vi "tcp connlimit test.vi"() -> ()   [LabVIEW 2015]
uses:
  connection/connection maintainer.lvclass
  client/connection client.lvclass/connection client.ctl
  message/communicator message.lvclass
  message/communicator message.lvclass/communicator message.ctl
  communicator/communicator.lvclass/communicator.ctl
  client/prepare client.vi
  server/prepare server.vi
  TCP/TCP server.lvclass
  TCP client/TCP client.lvclass
  communicator/communicator.lvclass
  <vilib>/ptbypt/NI_PtbyPt.lvlib
panel:
  in  "close s":bool
  in  "close c1":bool
  in  "close c2":bool
  in  "remake c 2":bool
  in  "CS 3":cluster{"ID":string, "data":string}
  in  "C to S 2":bool
  out "ClienQ 2":refnum<class "connection maintainer.lvclass">
  out "ClienT 2":timestamp
  out "data 5":variant
  out "ID 5":string
  out "data 3":variant
  out "ID 3":string
  out "data":variant
  out "ID":string
  out "Numeric":dbl
  in  "remake s":bool
  in  "remake c":bool
  in  "CS 2":cluster{"ID":string, "data":string}
  in  "CS":cluster{"ID":string, "data":string}
  in  "S to C":bool
  in  "C to S":bool
  in  "exits":bool
  out "ClienT":timestamp
  out "servT":timestamp
  out "servQ":refnum<class "connection maintainer.lvclass">
  out "ClienQ":refnum<class "connection maintainer.lvclass">
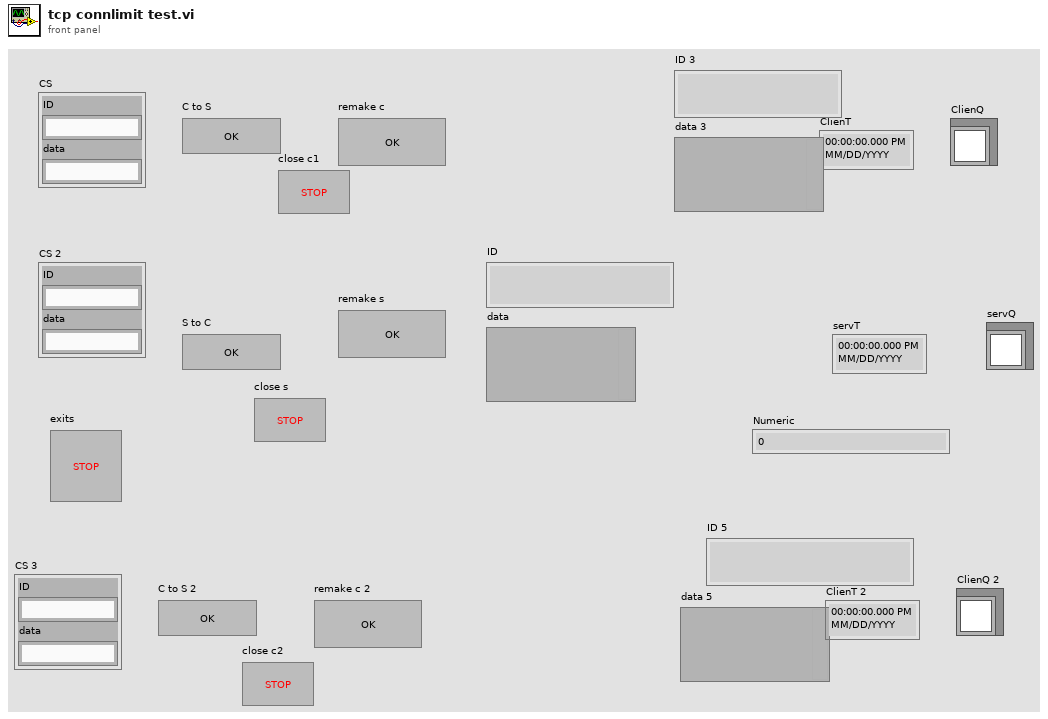
[diagram p1: front panel]
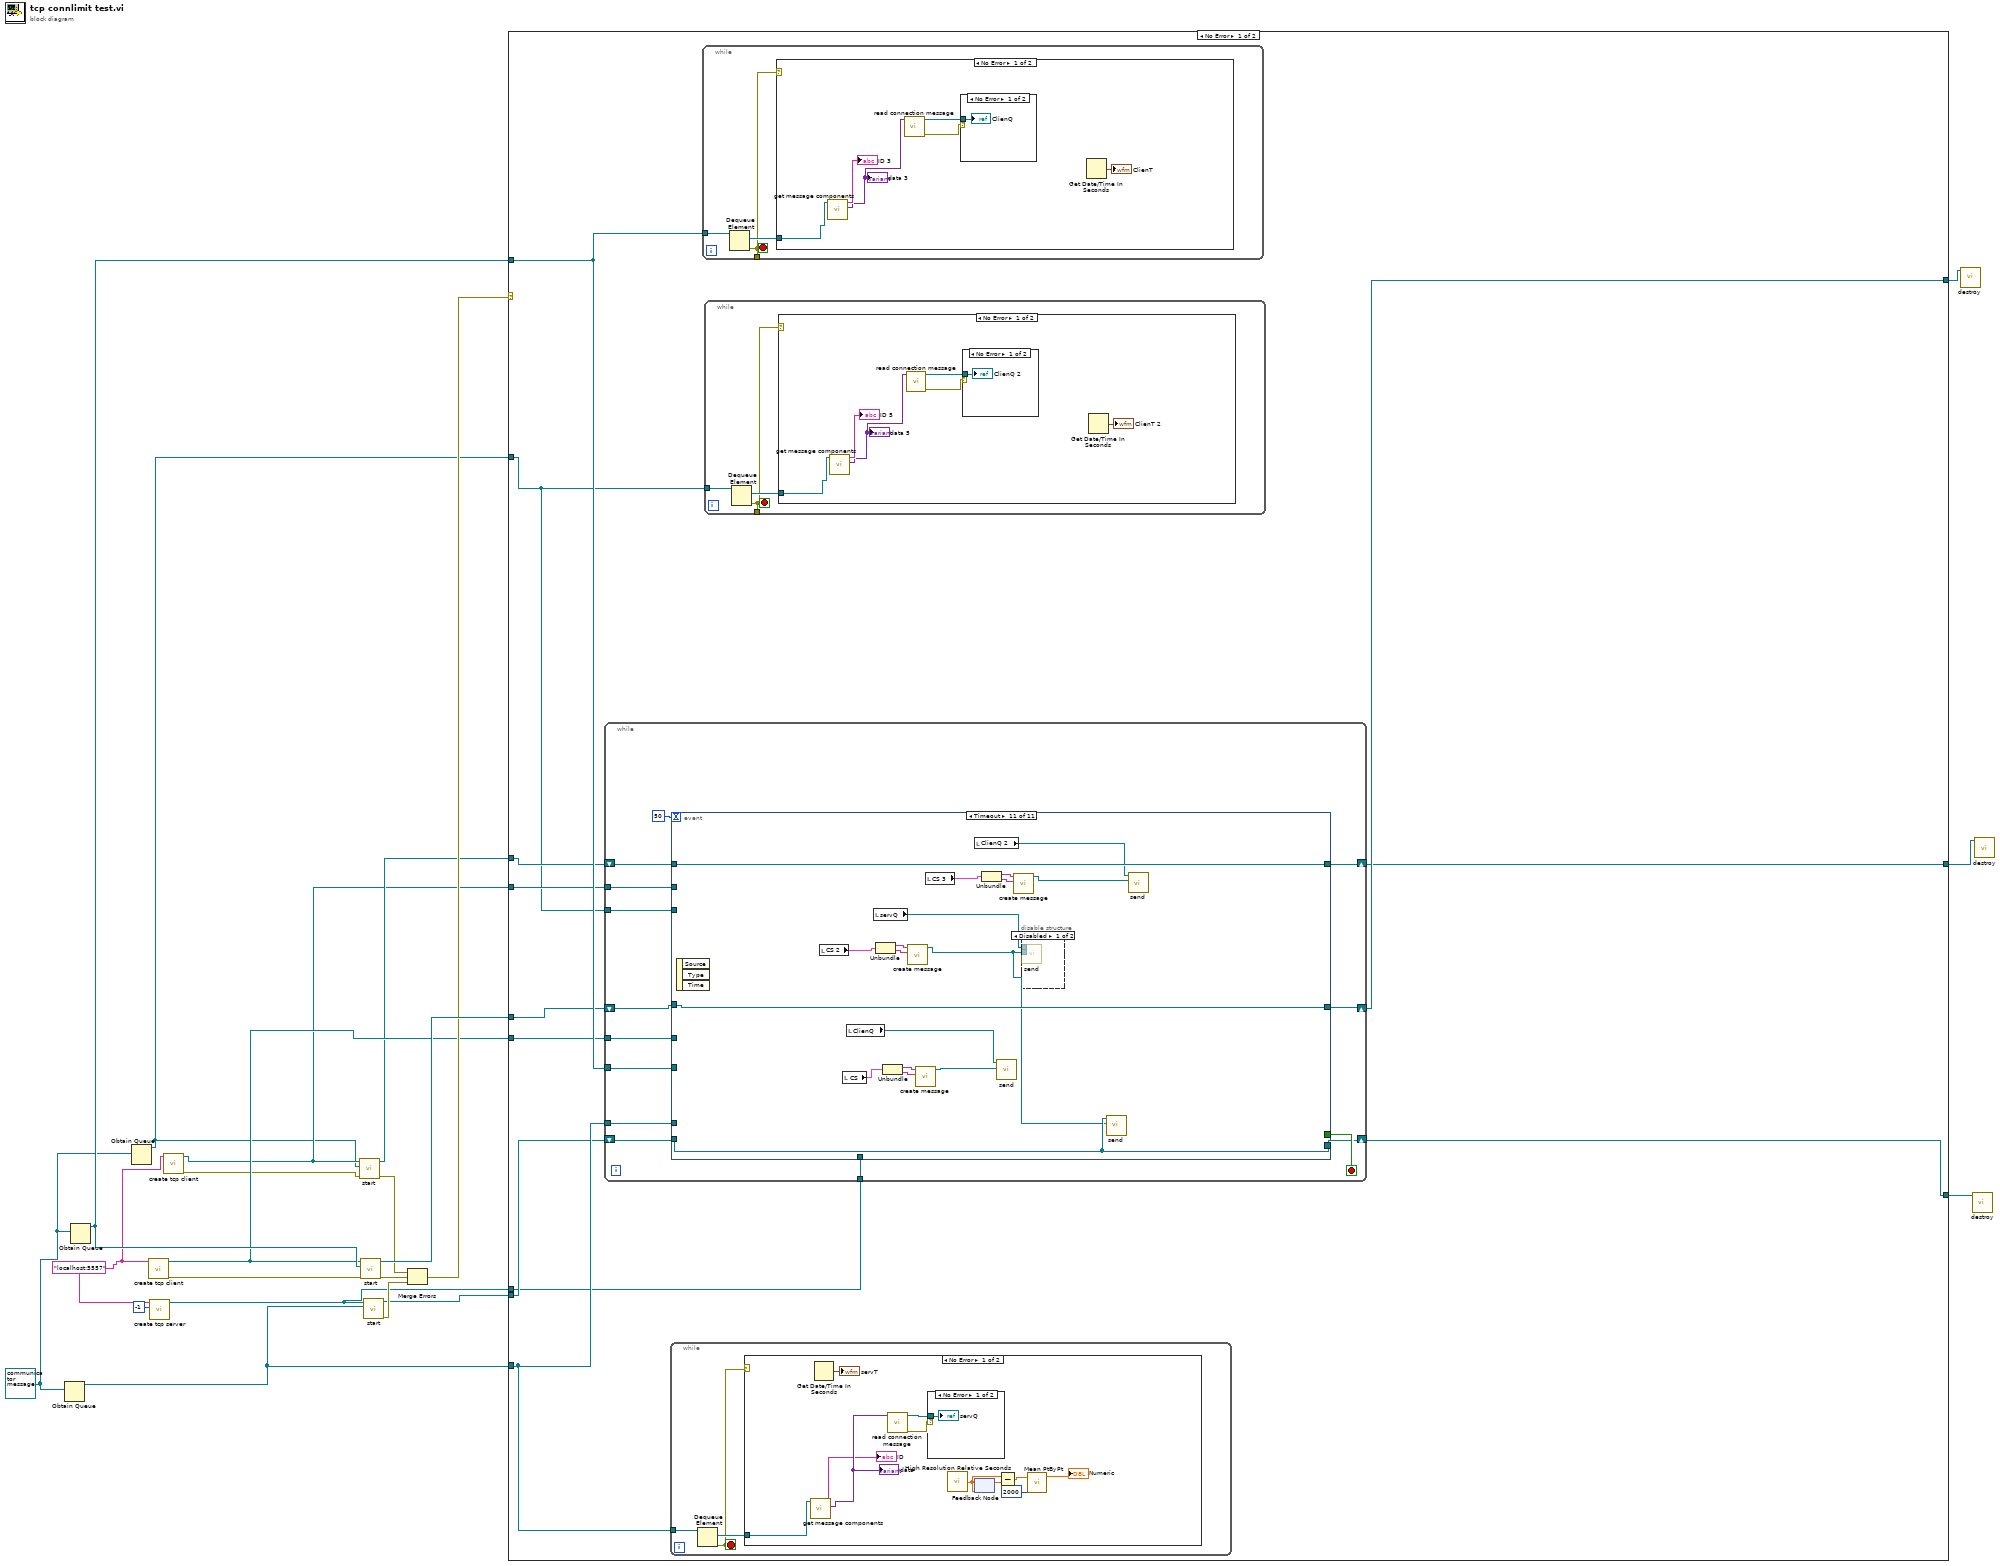
[diagram p0: block diagram]
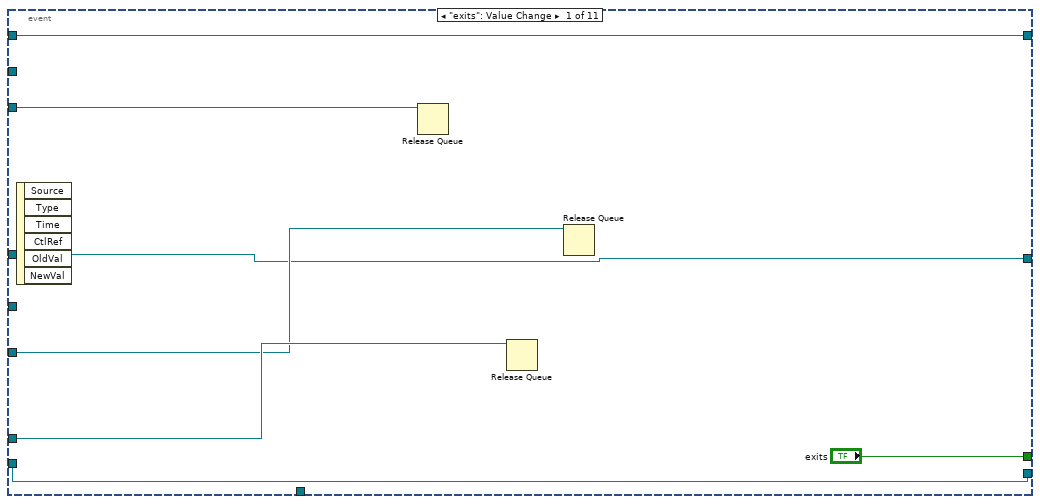
[diagram p4: hidden frame]
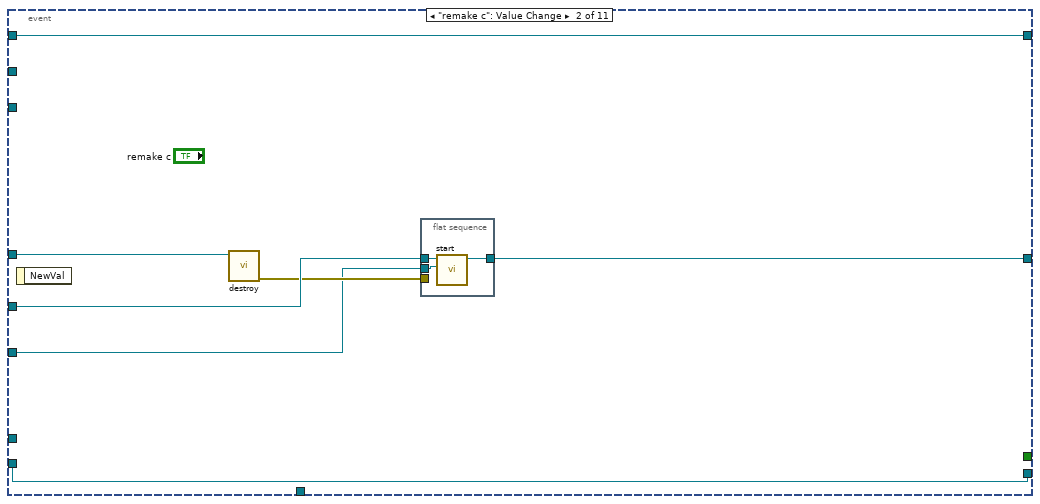
[diagram p5: hidden frame]
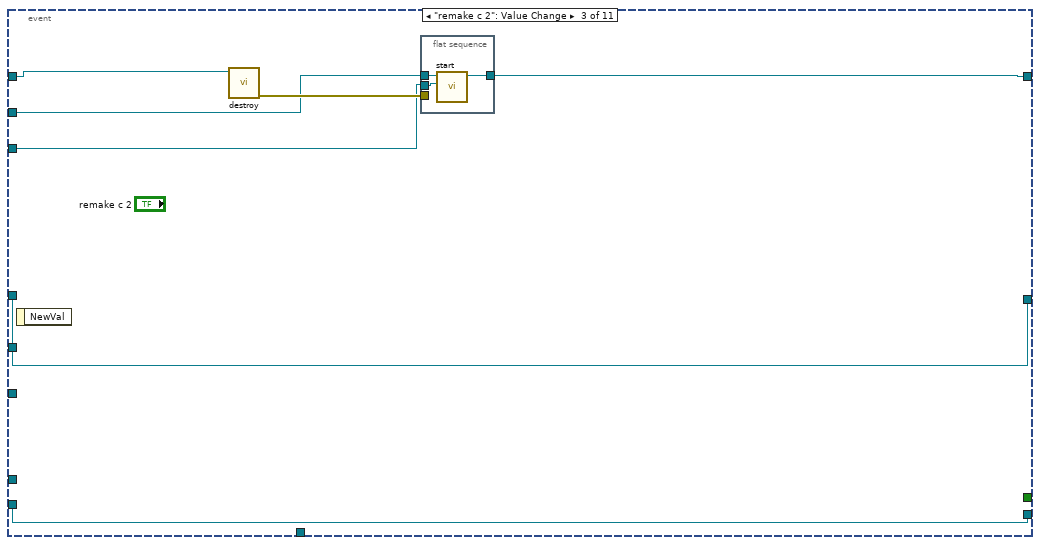
[diagram p6: hidden frame]
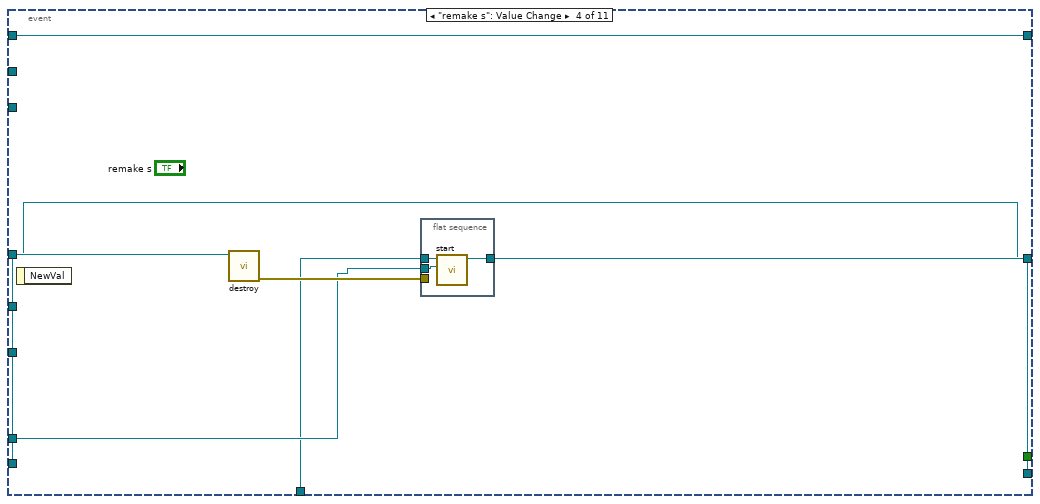
[diagram p7: hidden frame]
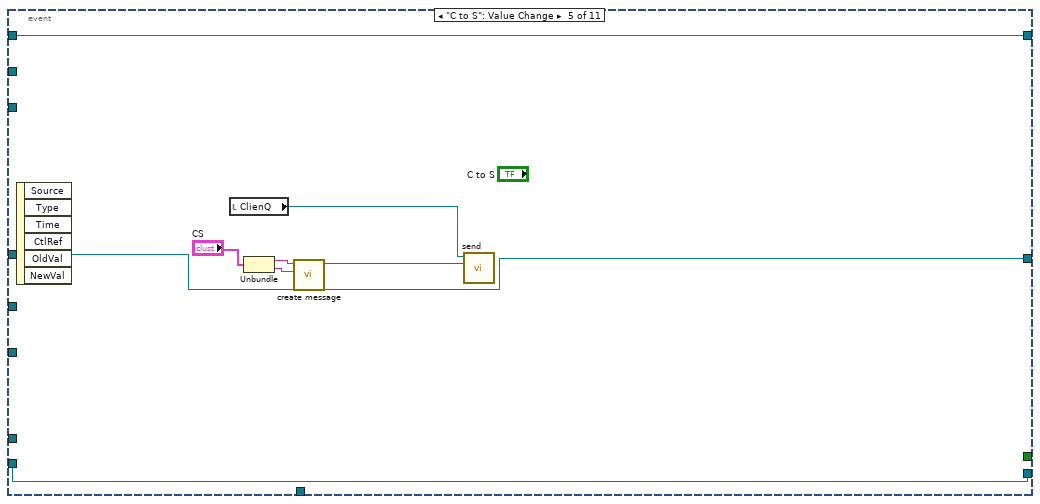
[diagram p8: hidden frame]
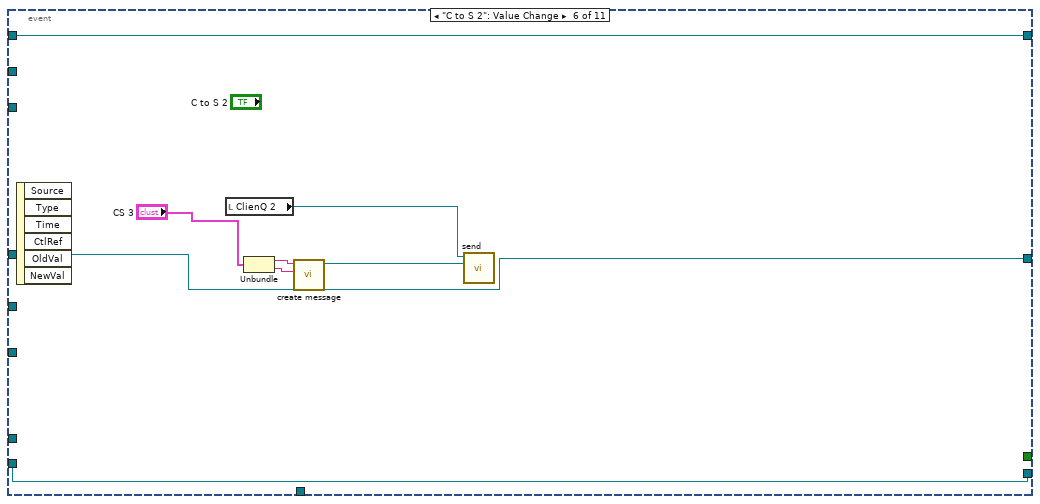
[diagram p9: hidden frame]
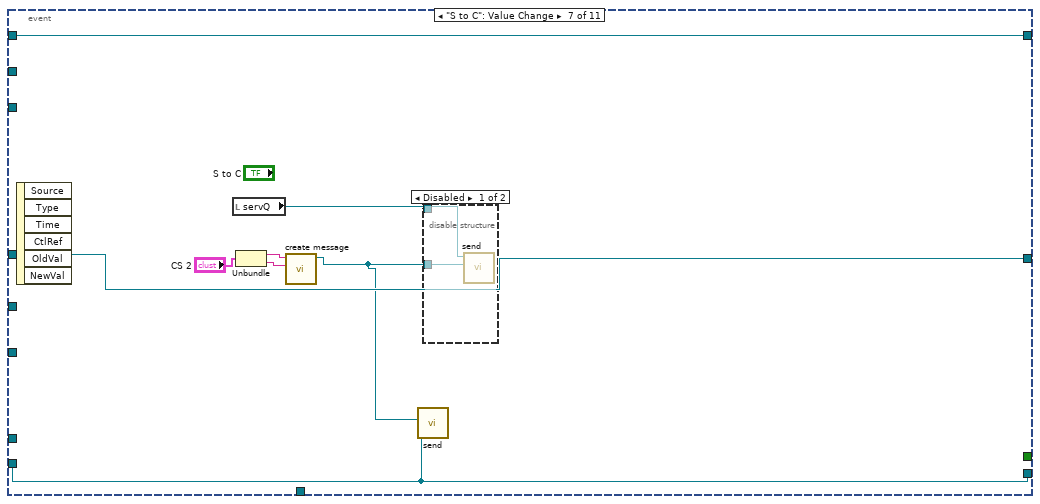
[diagram p10: hidden frame]
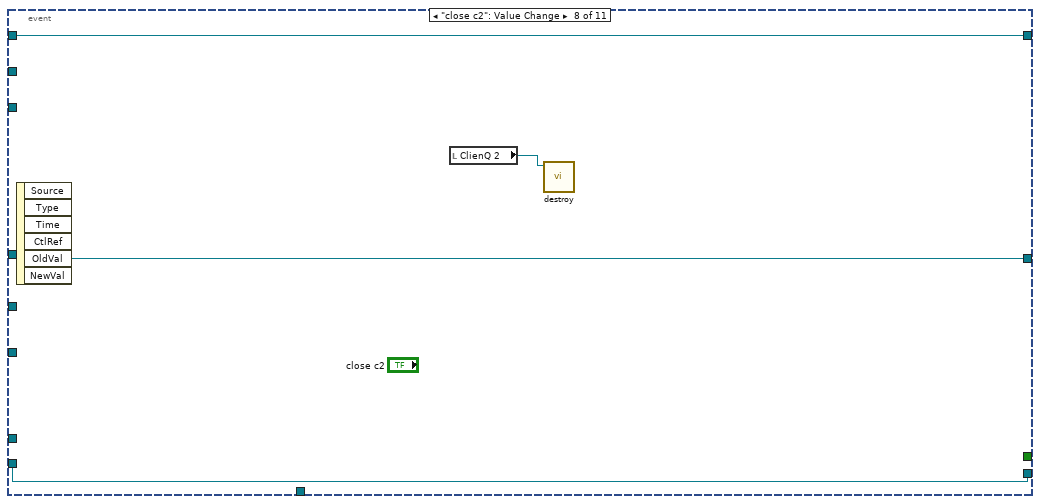
[diagram p12: hidden frame]
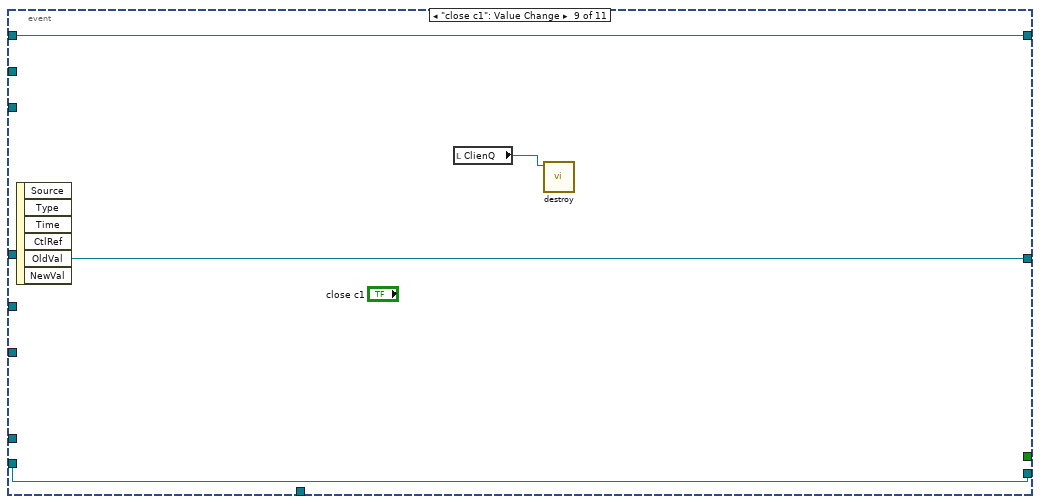
[diagram p13: hidden frame]
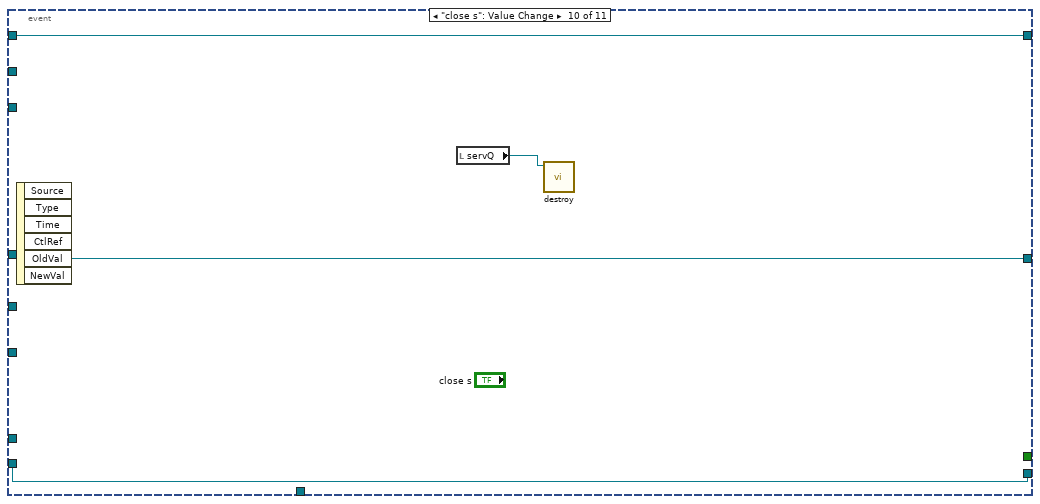
[diagram p14: hidden frame]
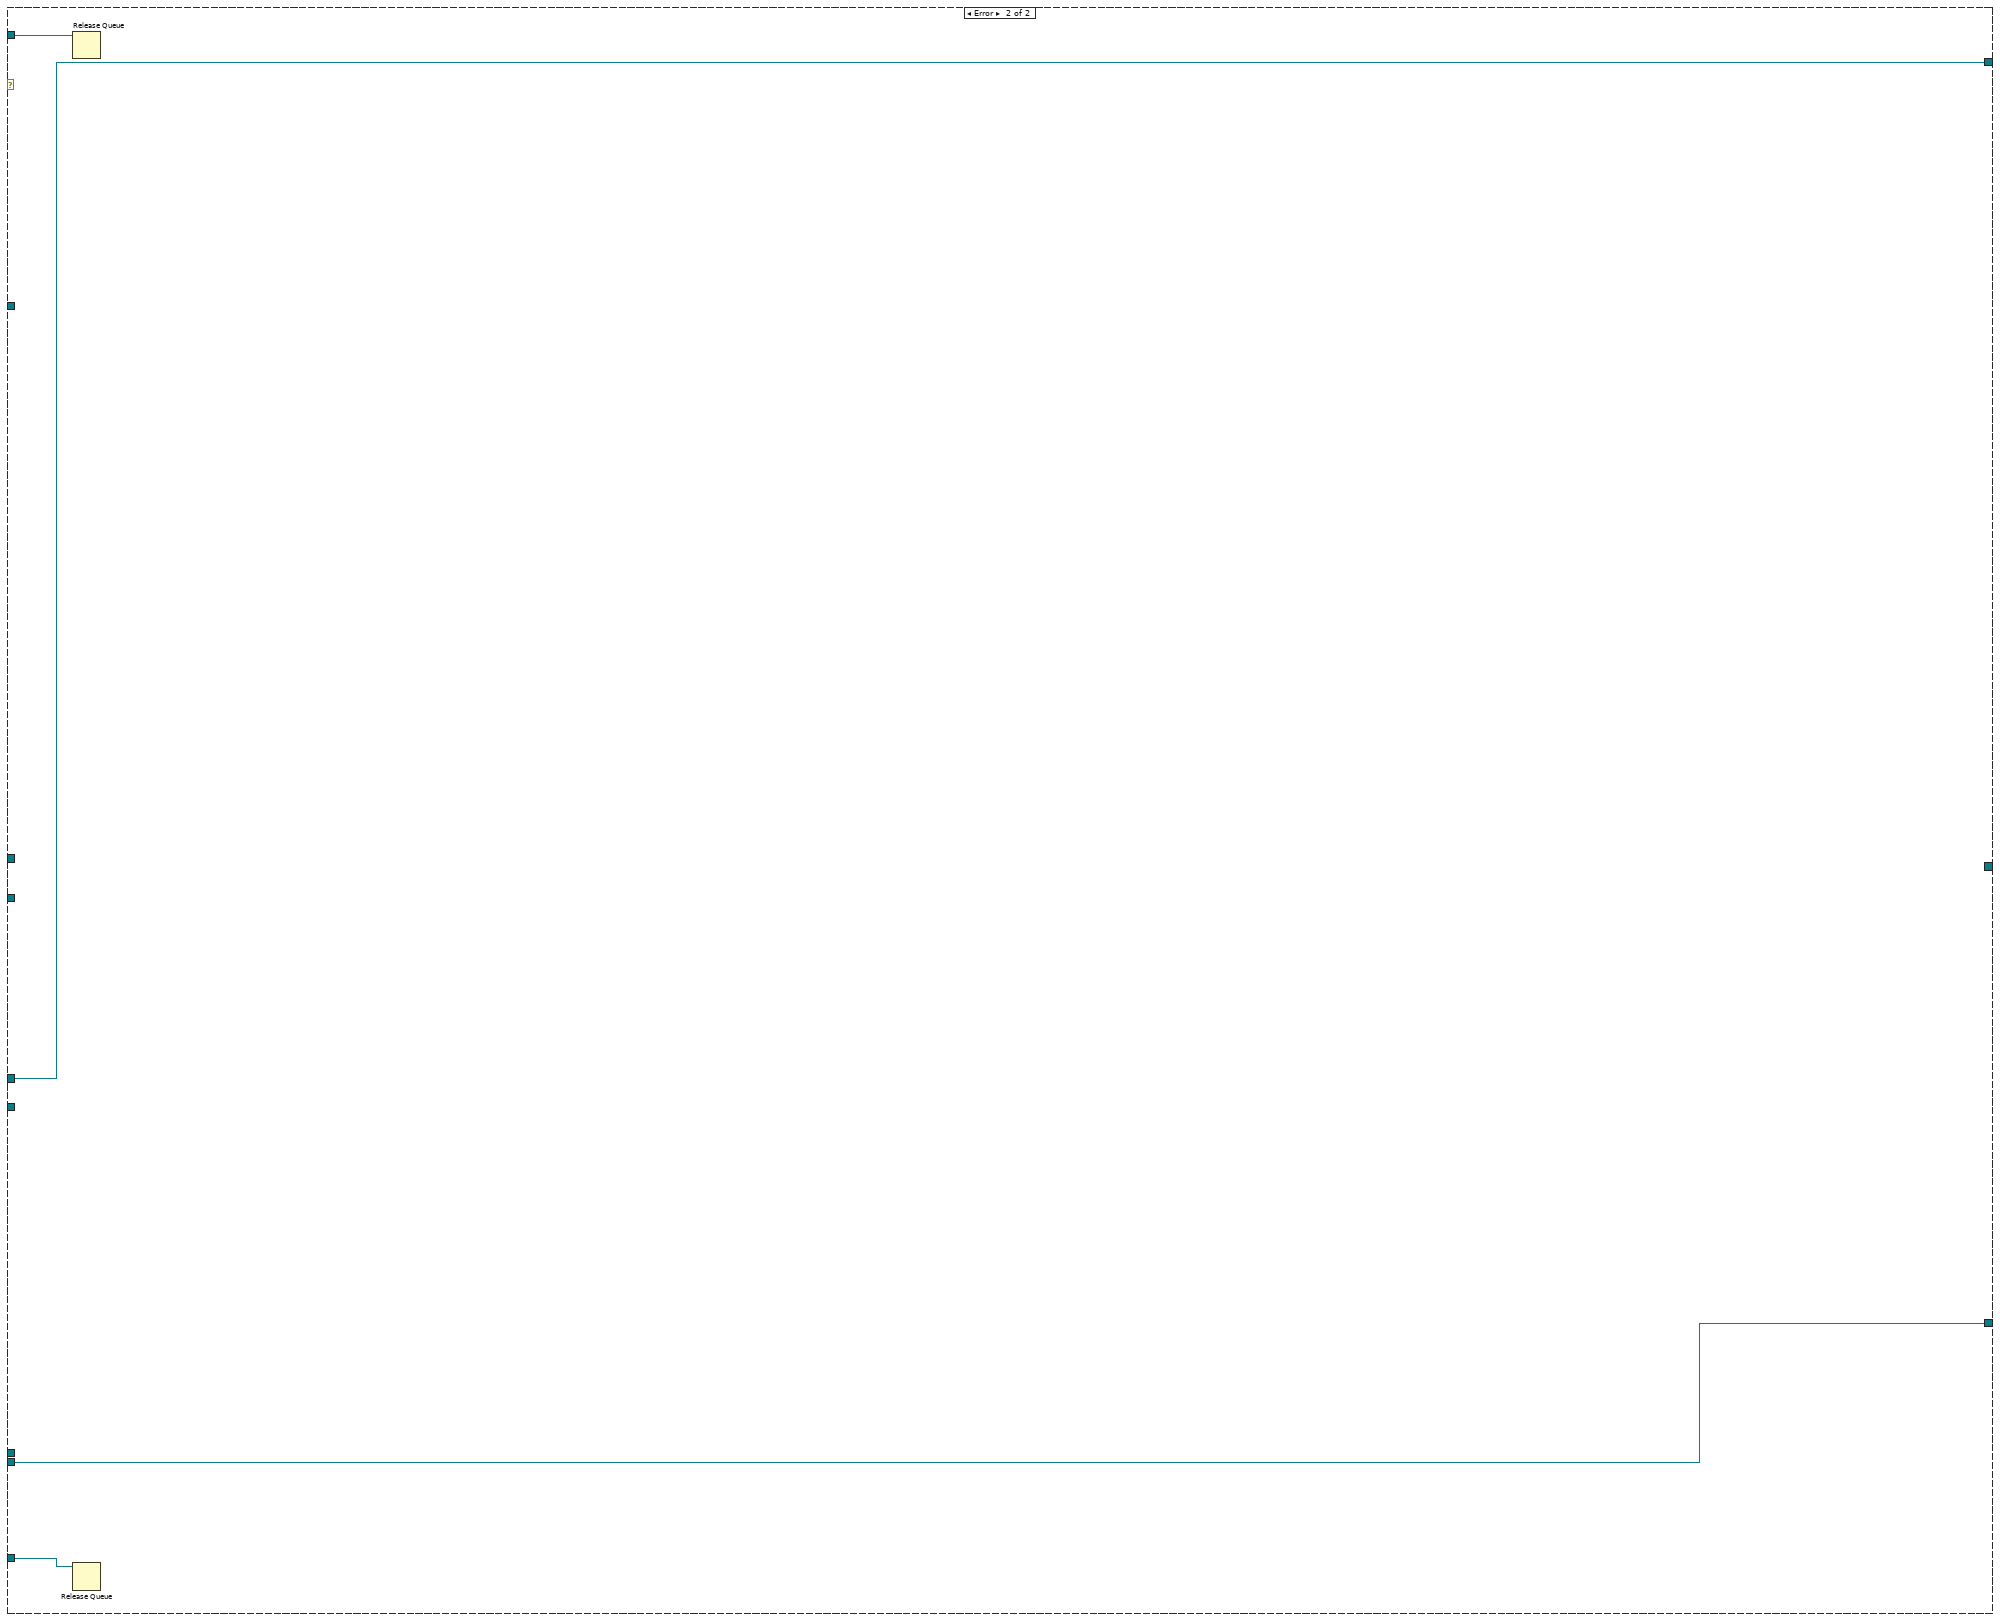
[diagram p20: hidden frame]
diagram:
  w9 = refnum<class "communicator message.lvclass"> refnum ("message")
  w5 = "localhost:5557" ("connection string")
  n1 = Obtain Queue(element data type=w9) -> (queue out=w14:refnum<queue>)  [unwired: 4 in, 2 out]
  n2 = Obtain Queue(element data type=w9) -> (queue out=w15:refnum<queue>)  [unwired: 4 in, 2 out]
  n3 = Obtain Queue(element data type=w9) -> (queue out=w3:refnum<queue>)  [unwired: 4 in, 2 out]
  n4 = call "create tcp client.vi"("conn string"=w5) -> ("error out"=w20:errorcluster, "TCP client out"=w11:refnum<class "TCP client.lvclass">)  [unwired: 9 in]
  n5 = call "create tcp server.vi"("max allowed"=-1, "conn string"=w5) -> ("TCP server out"=w10:refnum<class "TCP server.lvclass">)  [unwired: 8 in, 1 out]
  n6 = call "create tcp client.vi"("conn string"=w5) -> ("error out"=w8:errorcluster, "TCP client out"=w4:refnum<class "TCP client.lvclass">)  [unwired: 9 in]
  n7 = call-dynamic "start.vi"("error in"=w8, "queue to parent"=w3, "communicator in"=w4) -> ("error out"=w7:errorcluster, "communicator out"=w6:refnum<class "TCP client.lvclass">)  [unwired: 7 in]
  n8 = call-dynamic "start.vi"("error in"=w20, "queue to parent"=w15, "communicator in"=w11) -> ("error out"=w18:errorcluster, "communicator out"=w19:refnum<class "TCP client.lvclass">)  [unwired: 7 in]
  n9 = call-dynamic "start.vi"("queue to parent"=w14, "communicator in"=w10) -> ("error out"=w16:errorcluster, "communicator out"=w13:refnum<class "TCP server.lvclass">)  [unwired: 8 in]
  n10 = Merge Errors(w7, w18, w16) -> (w17:errorcluster)
  n11 = case shown="No Error" w17 {
    tunnel: [w26 w180] -> w21
    tunnel: w15 -> [w32 w181]
    tunnel: w19 -> [w31 w180]
    tunnel: w14 -> [w33 w179]
    tunnel: w13 -> [w29 w178]
    tunnel: [w27 w178] -> w12
    tunnel: w11 -> [w30 _]
    tunnel: w10 -> [w28 _]
    tunnel: w6 -> [w25 _]
    tunnel: w3 -> [w22 _]
    tunnel: w4 -> [w24 _]
    tunnel: [w23 _] -> w2
    frame No Error {
      n12 = while {
        tunnel: w33 -> [w56]
        tunnel: w32 -> [w55]
        tunnel: w30 -> [w53]
        tunnel: w28 -> [w51]
        shift-right: [w50] -> w27
        shift-left: w29 -> [w52]
        shift-right: [w49] -> w26
        shift-left: w31 -> [w54]
        shift-right: [w47] -> w23
        shift-left: w25 -> [w46]
        tunnel: w24 -> [w45]
        tunnel: w22 -> [w44]
        stop <- w57 stop-if-true
        n13 = event shown="[10] Timeout" {
          selector: _ -> [_ _ _ _ _ _ _ _ _ _ _]
          dyn-events: _ -> [_ _ _ _ _ _ _ _ _ _ _]
          timeout: 50 -> [_ _ _ _ _ _ _ _ _ _ _]
          tunnel: ["exits" _ _ _ _ _ _ _ _ _ _] -> w57
          tunnel: w56 -> [w63 _ _ w89 _ _ _ _ _ _ _]
          tunnel: w55 -> [w62 w68 _ _ _ _ _ _ _ _ _]
          tunnel: w54 -> [w60 w71 w76 w86 w100 w108 w117 w123 w127 w131 w150]
          tunnel: w53 -> [_ w70 _ _ _ _ _ _ _ _ _]
          tunnel: w52 -> [w61 w67 w80 w90 w101 w109 w112 w124 w128 w132 w134]
          tunnel: w51 -> [_ _ _ w88 _ _ _ _ _ _ _]
          tunnel: [w61 w67 w80 w87 w101 w109 w112 w124 w128 w132 w134] -> w50
          tunnel: [w60 w66 w76 w86 w100 w108 w117 w123 w127 w131 w150] -> w49
          tunnel: [w59 w65 w77 w85 w96 w104 w113 w122 w126 w130 w149] -> w47
          tunnel: w46 -> [w59 w65 w79 w85 w96 w104 w113 w122 w126 w130 w149]
          tunnel: w45 -> [_ _ w78 _ _ _ _ _ _ _ _]
          tunnel: w44 -> [w58 _ w75 _ _ _ _ _ _ _ _]
          event "exits": Value Change {
            n14 = event-data() -> ()  [unwired: 1 in, 6 out]
            n15 = Release Queue(queue=w58) -> ()  [unwired: 2 in, 3 out]
            n16 = Release Queue(queue=w63) -> ()  [unwired: 2 in, 3 out]
            n17 = Release Queue(queue=w62) -> ()  [unwired: 2 in, 3 out]
          }
          event "remake c": Value Change {
            n18 = event-data() -> ()  [unwired: 1 in, 1 out]
            n19 = call-dynamic "destroy.vi"("communicator in"=w71) -> ("error out"=w69:errorcluster)  [unwired: 10 in]
            n20 = flat-sequence {
              tunnel: w70 -> [w74]
              tunnel: w69 -> [_]
              tunnel: w68 -> [w73]
              tunnel: [w72] -> w66
              frame #0 {
                n21 = call-dynamic "start.vi"("queue to parent"=w73, "communicator in"=w74) -> ("communicator out"=w72:refnum<class "TCP client.lvclass">)  [unwired: 8 in, 1 out]
              }
            }
          }
          event "remake c 2": Value Change {
            n22 = event-data() -> ()  [unwired: 1 in, 1 out]
            n23 = call-dynamic "destroy.vi"("communicator in"=w79) -> ("error out"=w81:errorcluster)  [unwired: 10 in]
            n24 = flat-sequence {
              tunnel: w78 -> [w84]
              tunnel: w81 -> [_]
              tunnel: w75 -> [w83]
              tunnel: [w82] -> w77
              frame #0 {
                n25 = call-dynamic "start.vi"("queue to parent"=w83, "communicator in"=w84) -> ("communicator out"=w82:refnum<class "TCP client.lvclass">)  [unwired: 8 in, 1 out]
              }
            }
          }
          event "remake s": Value Change {
            n26 = event-data() -> ()  [unwired: 1 in, 1 out]
            n27 = call-dynamic "destroy.vi"("communicator in"=w90) -> ("error out"=w91:errorcluster)  [unwired: 10 in]
            n28 = flat-sequence {
              tunnel: w88 -> [w94]
              tunnel: w91 -> [_]
              tunnel: w89 -> [w93]
              tunnel: [w92] -> w87
              frame #0 {
                n29 = call-dynamic "start.vi"("queue to parent"=w93, "communicator in"=w94) -> ("communicator out"=w92:refnum<class "TCP server.lvclass">)  [unwired: 8 in, 1 out]
              }
            }
          }
          event "C to S": Value Change {
            n30 = event-data() -> ()  [unwired: 1 in, 6 out]
            n31 = local read "ClienQ"() -> (w102:refnum<class "connection maintainer.lvclass">)
            n32 = Unbundle("CS") -> ("ID"=w99:string, "data"=w98:string)
            n33 = call "create message.vi"("data"=w98, "ID"=w99) -> ("message"=w95:refnum<class "communicator message.lvclass">)  [unwired: 9 in]
            n34 = call "send.vi"("element"=w95, "communicator in"=w102) -> ()  [unwired: 9 in, 1 out]
          }
          event "C to S 2": Value Change {
            n35 = event-data() -> ()  [unwired: 1 in, 6 out]
            n36 = local read "ClienQ 2"() -> (w110:refnum<class "connection maintainer.lvclass">)
            n37 = Unbundle("CS 3") -> ("ID"=w107:string, "data"=w106:string)
            n38 = call "create message.vi"("data"=w106, "ID"=w107) -> ("message"=w103:refnum<class "communicator message.lvclass">)  [unwired: 9 in]
            n39 = call "send.vi"("element"=w103, "communicator in"=w110) -> ()  [unwired: 9 in, 1 out]
          }
          event "S to C": Value Change {
            n40 = event-data() -> ()  [unwired: 1 in, 6 out]
            n41 = local read "servQ"() -> (w118:refnum<class "connection maintainer.lvclass">)
            n42 = Unbundle("CS 2") -> ("ID"=w116:string, "data"=w115:string)
            n43 = call "create message.vi"("data"=w115, "ID"=w116) -> ("message"=w111:refnum<class "communicator message.lvclass">)  [unwired: 9 in]
            n44 = call "send.vi"("element"=w111, "communicator in"=w112) -> ()  [unwired: 9 in, 1 out]
            n45 = disable-structure shown="Disabled" {
              disable-tunnel: w118 -> [w120 _]
              disable-tunnel: w111 -> [w119 _]
              frame Disabled {
                n46 = call "send.vi"("element"=w119, "communicator in"=w120) -> ()  [unwired: 9 in, 1 out]
              }
              frame Enabled {
              }
            }
          }
          event "close c2": Value Change {
            n47 = event-data() -> ()  [unwired: 1 in, 6 out]
            n48 = local read "ClienQ 2"() -> (w121:refnum<class "connection maintainer.lvclass">)
            n49 = call-dynamic "destroy.vi"("communicator in"=w121) -> ()  [unwired: 10 in, 1 out]
          }
          event "close c1": Value Change {
            n50 = event-data() -> ()  [unwired: 1 in, 6 out]
            n51 = local read "ClienQ"() -> (w125:refnum<class "connection maintainer.lvclass">)
            n52 = call-dynamic "destroy.vi"("communicator in"=w125) -> ()  [unwired: 10 in, 1 out]
          }
          event "close s": Value Change {
            n53 = event-data() -> ()  [unwired: 1 in, 6 out]
            n54 = local read "servQ"() -> (w129:refnum<class "connection maintainer.lvclass">)
            n55 = call-dynamic "destroy.vi"("communicator in"=w129) -> ()  [unwired: 10 in, 1 out]
          }
          event Timeout {
            n56 = event-data() -> ()  [unwired: 1 in, 3 out]
            n57 = local read "CS 2"() -> (w148:cluster{"ID":string, "data":string})
            n58 = local read "CS"() -> (w141:cluster{"ID":string, "data":string})
            n59 = local read "ClienQ"() -> (w144:refnum<class "connection maintainer.lvclass">)
            n60 = local read "servQ"() -> (w147:refnum<class "connection maintainer.lvclass">)
            n61 = Unbundle(w148) -> ("ID"=w146:string, "data"=w145:string)
            n62 = Unbundle(w141) -> ("ID"=w143:string, "data"=w142:string)
            n63 = call "create message.vi"("data"=w145, "ID"=w146) -> ("message"=w133:refnum<class "communicator message.lvclass">)  [unwired: 9 in]
            n64 = call "create message.vi"("data"=w142, "ID"=w143) -> ("message"=w140:refnum<class "communicator message.lvclass">)  [unwired: 9 in]
            n65 = local read "CS 3"() -> (w135:cluster{"ID":string, "data":string})
            n66 = local read "ClienQ 2"() -> (w136:refnum<class "connection maintainer.lvclass">)
            n67 = Unbundle(w135) -> ("ID"=w138:string, "data"=w139:string)
            n68 = call "send.vi"("element"=w140, "communicator in"=w144) -> ()  [unwired: 9 in, 1 out]
            n69 = call "create message.vi"("data"=w139, "ID"=w138) -> ("message"=w137:refnum<class "communicator message.lvclass">)  [unwired: 9 in]
            n70 = disable-structure shown="Disabled" {
              disable-tunnel: w147 -> [w152 _]
              disable-tunnel: w133 -> [w151 _]
              frame Disabled {
                n71 = call "send.vi"("element"=w151, "communicator in"=w152) -> ()  [unwired: 9 in, 1 out]
              }
              frame Enabled {
              }
            }
            n72 = call "send.vi"("element"=w133, "communicator in"=w134) -> ()  [unwired: 9 in, 1 out]
            n73 = call "send.vi"("element"=w137, "communicator in"=w136) -> ()  [unwired: 9 in, 1 out]
          }
        }
      }
      n74 = while {
        tunnel: w33 -> [w155]
        stop <- w153 stop-if-true
        n75 = Dequeue Element(queue=w155) -> (element=w154:refnum<class "communicator message.lvclass">, error out=w153:errorcluster)  [unwired: 2 in, 2 out]
        n76 = case shown="No Error" w153 {
          tunnel: w154 -> [w156 _]
          frame No Error {
            n77 = call "get message components.vi"("message"=w156) -> ("data"=w158:variant, "ID"=→"ID":string)  [unwired: 9 in]
            "data" <- w158
            n78 = Get Date/Time In Seconds() -> (seconds since 1Jan1904=→"servT":timestamp)
            n79 = call "read connection message.vi"("data"=w158) -> ("error out"=w165:errorcluster, "conn"=w166:refnum<class "connection maintainer.lvclass">)  [unwired: 9 in]
            n80 = case shown="No Error" w165 {
              tunnel: w166 -> [w167 _]
              frame No Error {
                "servQ" <- w167
              }
              frame Error {
              }
            }
            n81 = call <vilib>:"High Resolution Relative Seconds.vi"() -> ("relative seconds"=w162:dbl)
            n82 = feedback-in #1(w162) -> ()
            n83 = feedback #1(w162) -> (w163:dbl)
            n84 = Subtract(x=w162, y=w163) -> (x-y=w161:dbl)
            n85 = call <vilib>:"Mean PtByPt.vi"("x"=w161, "sample length"=2000) -> ("mean"=→"Numeric":dbl)  [unwired: 2 in, 1 out]
          }
          frame Error {
          }
        }
      }
      n86 = while {
        tunnel: w32 -> [w170]
        tunnel: [w168] -> _
        stop <- w168 stop-if-true
        n87 = Dequeue Element(queue=w170) -> (element=w169:refnum<class "communicator message.lvclass">, error out=w168:errorcluster)  [unwired: 2 in, 2 out]
        n88 = case shown="No Error" w168 {
          tunnel: w169 -> [w172 _]
          frame No Error {
            n89 = call "get message components.vi"("message"=w172) -> ("data"=w171:variant, "ID"=→"ID 3":string)  [unwired: 9 in]
            "data 3" <- w171
            n90 = call "read connection message.vi"("data"=w171) -> ("error out"=w175:errorcluster, "conn"=w176:refnum<class "connection maintainer.lvclass">)  [unwired: 9 in]
            n91 = case shown="No Error" w175 {
              tunnel: w176 -> [w177 _]
              frame No Error {
                "ClienQ" <- w177
              }
              frame Error {
              }
            }
            n92 = Get Date/Time In Seconds() -> (seconds since 1Jan1904=→"ClienT":timestamp)
          }
          frame Error {
          }
        }
      }
      n93 = while {
        tunnel: w22 -> [w36]
        tunnel: [w34] -> _
        stop <- w34 stop-if-true
        n94 = Dequeue Element(queue=w36) -> (element=w35:refnum<class "communicator message.lvclass">, error out=w34:errorcluster)  [unwired: 2 in, 2 out]
        n95 = case shown="No Error" w34 {
          tunnel: w35 -> [w38 _]
          frame No Error {
            n96 = call "get message components.vi"("message"=w38) -> ("data"=w37:variant, "ID"=→"ID 5":string)  [unwired: 9 in]
            "data 5" <- w37
            n97 = call "read connection message.vi"("data"=w37) -> ("error out"=w41:errorcluster, "conn"=w42:refnum<class "connection maintainer.lvclass">)  [unwired: 9 in]
            n98 = case shown="No Error" w41 {
              tunnel: w42 -> [w43 _]
              frame No Error {
                "ClienQ 2" <- w43
              }
              frame Error {
              }
            }
            n99 = Get Date/Time In Seconds() -> (seconds since 1Jan1904=→"ClienT 2":timestamp)
          }
          frame Error {
          }
        }
      }
    }
    frame Error {
      n100 = Release Queue(queue=w181) -> ()  [unwired: 2 in, 3 out]
      n101 = Release Queue(queue=w179) -> ()  [unwired: 2 in, 3 out]
    }
  }
  n102 = call-dynamic "destroy.vi"("communicator in"=w21) -> ()  [unwired: 10 in, 1 out]
  n103 = call-dynamic "destroy.vi"("communicator in"=w12) -> ()  [unwired: 10 in, 1 out]
  n104 = call-dynamic "destroy.vi"("communicator in"=w2) -> ()  [unwired: 10 in, 1 out]
